vi "FPGA Acknowledge IRQs.vi"(8 "error in (no error)":errorcluster, 10 "IRQs":u32[](array[numeric]), 11 "FPGA Session In":refnum<class "FPGA Interface Base.lvclass">) -> (0 "error out":errorcluster, 3 "FPGA Session Out":refnum<class "FPGA Interface Base.lvclass">)   [LabVIEW 2010, in "FPGA Interface Base.lvclass"]
doc: "Acknowledges an IRQ or set of IRQs."
uses:
  <userlib>/_FPGA Interface Advanced Tools/FPGA Interface Base/FPGA Interface Base.lvclass
  <userlib>/_FPGA Interface Advanced Tools/FPGA Interface Base/Accessors/FPGA Read Session.vi
  <vilib>/Utility/error.llb/Error Cluster From Error Code.vi
  <userlib>/_FPGA Interface Advanced Tools/FPGA Interface Wrapper/FPGA Interface Wrapper.lvlib
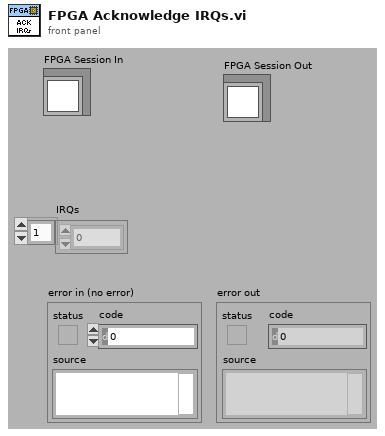
[diagram p1: front panel]
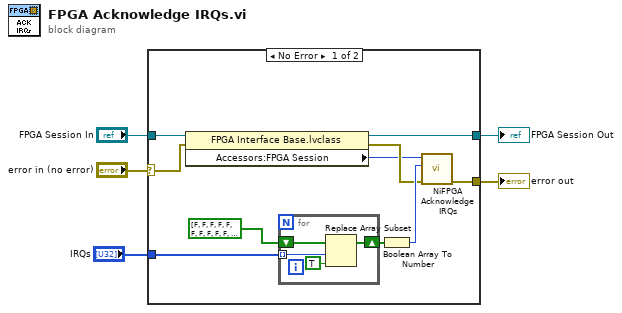
[diagram p0: block diagram]
diagram:
  n1 = case shown="No Error" "error in (no error)" {
    selector: "error in (no error)" -> [w10 w21]
    tunnel: [w7 w21] -> w2
    tunnel: [w6 w20] -> w4
    tunnel: "FPGA Session In" -> [w11 w20]
    tunnel: "IRQs" -> [w13 _]
    frame No Error {
      n2 = property class="FPGA Interface Base.lvclass"(reference=w11, error in=w10) -> (reference out=w6:refnum<class "FPGA Interface Base.lvclass">, error out=w9:errorcluster, "Accessors:FPGA Session"=w8:u32)
      n3 = for {
        tunnel: w13 -> [w18] mode=indexing
        shift-right: [w16] -> w15
        shift-left: bool[] [FALSE, FALSE, FALSE, FALSE, FALSE, FALSE, FALSE, FALSE, FALSE, FALSE, FALSE, FALSE, FALSE, FALSE, FALSE, FALSE, FALSE, FALSE, FALSE, FALSE, FALSE, FALSE, FALSE, FALSE, FALSE, FALSE, FALSE, FALSE, FALSE, FALSE, FALSE, FALSE] -> [w19]
        n4 = Replace Array Subset(array=w19, new element=TRUE ("new element/subarray"), index=w18) -> (w16:bool[])
      }
      n5 = Boolean Array To Number(Boolean array=w15) -> (number=w12:u32)
      n6 = call <userlib>:"NiFPGA Acknowledge IRQs.vi"("error in (no error)"=w9, "IRQs"=w12, "Session In"=w8) -> ("error out"=w7:errorcluster)  [unwired: 7 in, 1 out]
    }
    frame Error {
    }
  }
  "error out" <- w2
  "FPGA Session Out" <- w4
